vi "Stop All (User Event)- FGV.vi"(8 "error in":errorcluster, 10 "Action":T1=enum."Destroy") -> (0 "error out":errorcluster, 3 "User event ref":refnum<user-event>)   [LabVIEW 2018, in "Common.lvlib"]
doc: "Admin for user event which stops all modules."
uses:
  Common.lvlib
  ctl/Stop All - Action.ctl
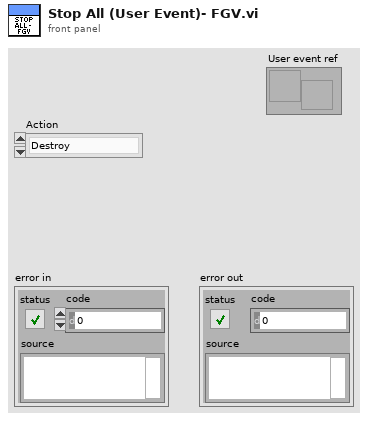
[diagram p1: front panel]
types:
  T1 = typedef "Common.lvlib/Stop All - Action.ctl" = enum16{"Create", "Fire", "Get", "Destroy"}
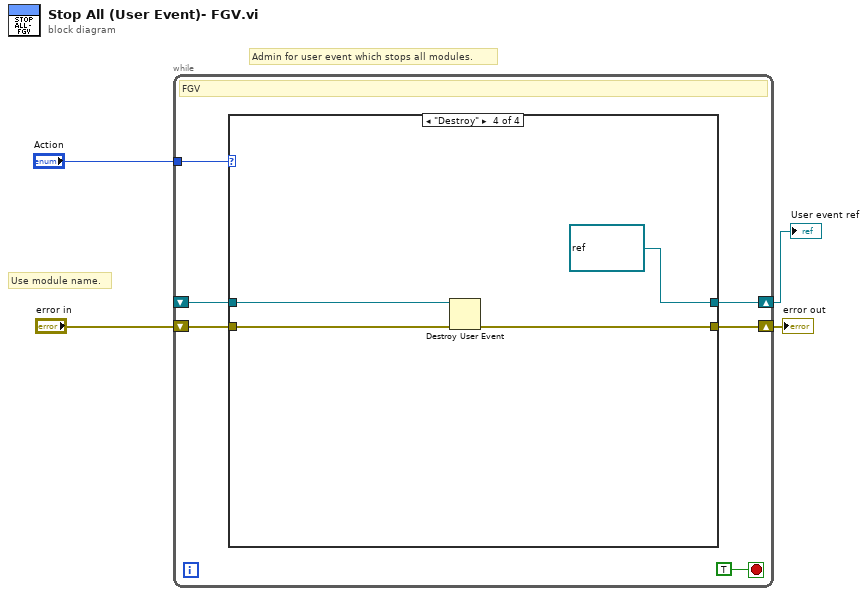
[diagram p0: block diagram]
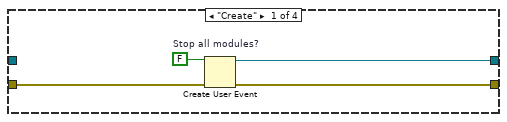
[diagram p2: hidden frame]
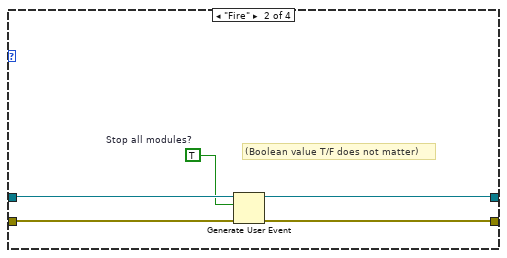
[diagram p3: hidden frame]
diagram:
  # "Admin for user event which stops all modules."
  # "Use module name."
  n1 = while {
    tunnel: "Action" -> [w9]
    shift-right: [w8] -> w1
    shift-left: _ -> [w5]
    shift-right: [w7] -> w3
    shift-left: "error in" -> [w6]
    stop <- TRUE stop-if-true
    # "FGV"
    n2 = case shown="\"Destroy\"" w9 {
      tunnel: [w14 w17 w21 refnum<user-event> refnum ("Stop all modules?")] -> w8
      tunnel: [w13 w16 w20 w23] -> w7
      tunnel: w6 -> [w12 w18 w20 w24]
      tunnel: w5 -> [_ w19 w21 w25]
      frame "Create" {
        w11 = FALSE  # Stop all modules?
        n3 = Create User Event(user event datatype=w11, error in=w12) -> (user event=w14:refnum<user-event>, error out=w13:errorcluster)
      }
      frame "Fire" {
        w15 = TRUE  # Stop all modules?
        # "(Boolean value T/F does not matter)"
        n4 = Generate User Event(user event=w19, event data cluster=w15, error in=w18) -> (user event out=w17:refnum<user-event>, error out=w16:errorcluster)  [unwired: 1 in]
      }
      frame "Get", Default {
      }
      frame "Destroy" {
        n5 = Destroy User Event(user event=w25, error in=w24) -> (error out=w23:errorcluster)
      }
    }
  }
  "error out" <- w3
  "User event ref" <- w1
